vi "WriteToMeasArray.vi"(8 "error in (no error)":errorcluster, 10 "RoomAlert Device Reference":refnum<vi>, 11 "RoomAlert in":refnum<class "RoomAlert.lvclass">) -> (0 "error out":errorcluster, 3 "RoomAlert out":refnum<class "RoomAlert.lvclass">)   [LabVIEW 2018, in "SensorPlugins.lvlib" / "RoomAlert.lvclass"]
doc: "Updates to the measurement array all the values a user may measure from the RoomAlert."
uses:
  RoomAlert.lvclass
  TypeDefinitions/RoomAlertControls.ctl
panel:
  in  "Text Ring":u16(ring)
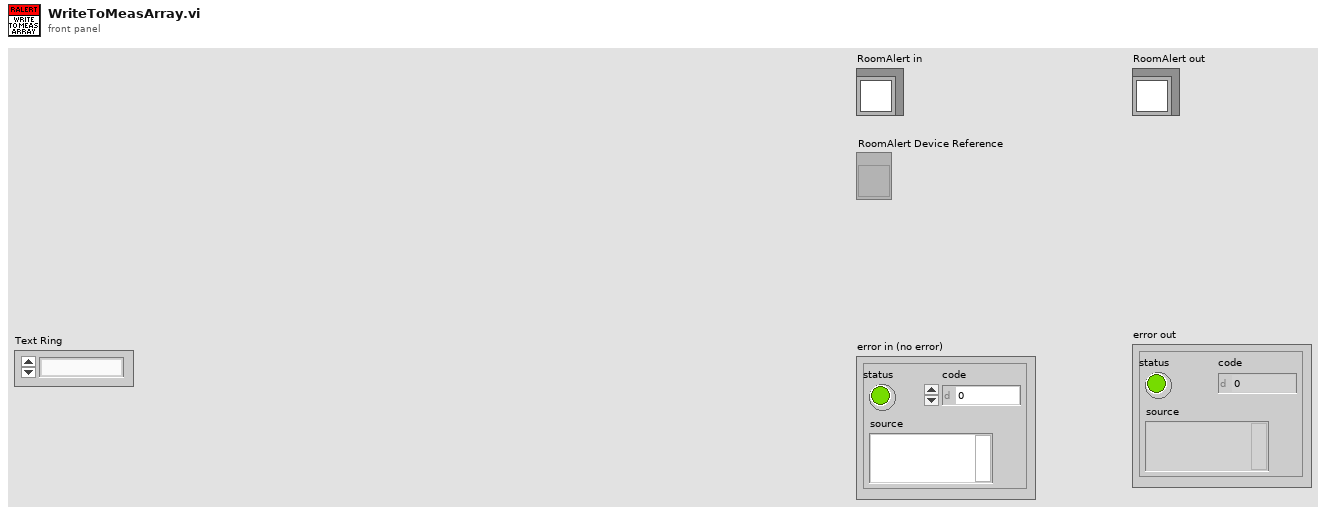
[diagram p1: front panel]
types:
  T1 = typedef "SensorPlugins.lvlib/RoomAlert.lvclass/MeasurementToRead.ctl" = cluster{"Type":string, "OID":string}[]
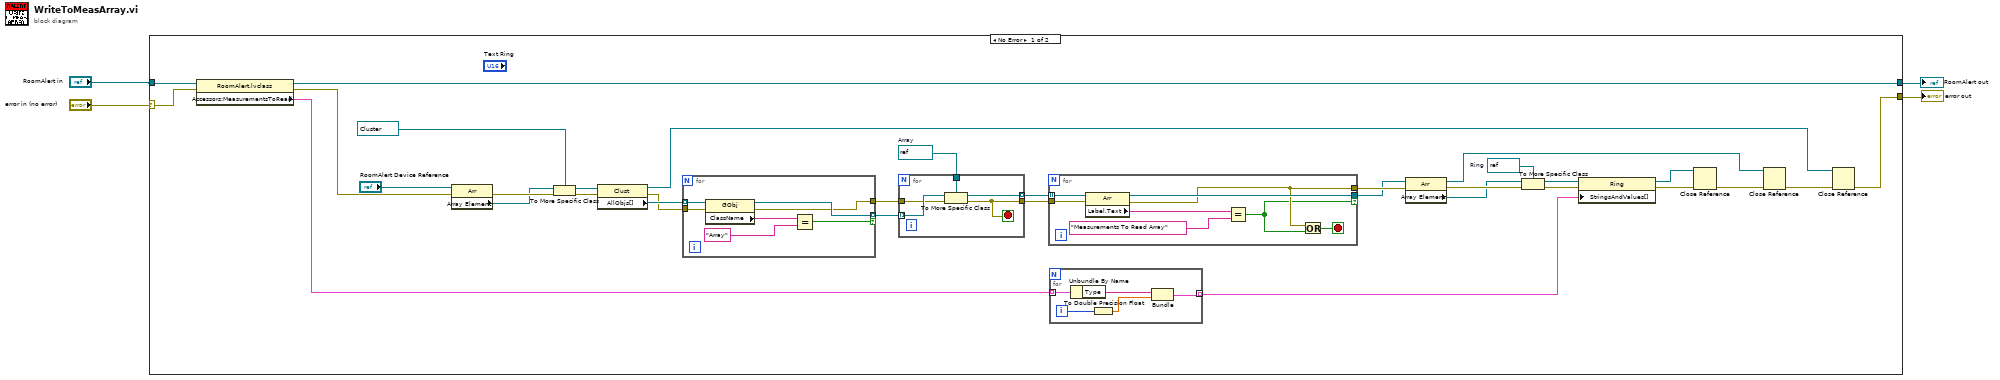
[diagram p0: block diagram]
diagram:
  n1 = case shown="No Error" "error in (no error)" {
    selector: "error in (no error)" -> [w36 w64]
    tunnel: [w19 w64] -> w1
    tunnel: [w35 w63] -> w2
    tunnel: "RoomAlert in" -> [w37 w63]
    frame No Error {
      w28 = refnum<vi> refnum  # Ring
      w8 = refnum<vi> refnum  # Array
      n2 = property class="RoomAlert.lvclass"(reference=w37, error in=w36) -> (reference out=w35:refnum<class "RoomAlert.lvclass">, error out=w34:errorcluster, "Accessors:MeasurementsToRead"=w14:T1)
      n3 = property class="Arr"(reference="RoomAlert Device Reference", error in=w34) -> (error out=w33:errorcluster, "Array Element"=w32:refnum<vi>)  [unwired: 1 out]
      n4 = To More Specific Class(target class=refnum<vi> refnum ("Text Ring"), reference=w32, error in=w33) -> (specific class reference=w29:refnum<vi>, error out=w30:errorcluster)
      n5 = property class="Clust"(reference=w29, error in=w30) -> (reference out=w16:refnum<vi>, error out=w11:errorcluster, "AllObjs[]"=w12:refnum<vi>[])
      n6 = for {
        tunnel: w12 -> [w44] mode=indexing
        tunnel: [w43] -> w9 mode=indexing if=w40
        tunnel: w11 -> [w41]
        tunnel: [w39] -> w10
        n7 = property class="GObj"(reference=w44, error in=w41) -> (reference out=w43:refnum<vi>, error out=w39:errorcluster, "ClassName"=w38:string)
        n8 = Equal?(x=w38, y="Array" ("ClassName")) -> (x = y?=w40:bool)
      }
      n9 = for {
        tunnel: w10 -> [w52]
        tunnel: w9 -> [w53] mode=indexing
        tunnel: w8 -> [w54]
        tunnel: [w51] -> w7 mode=indexing
        tunnel: [w50] -> w6
        stop <- w50 stop-if-true
        n10 = To More Specific Class(target class=w54, reference=w53, error in=w52) -> (specific class reference=w51:refnum<vi>, error out=w50:errorcluster)
      }
      n11 = for {
        tunnel: w7 -> [w62] mode=indexing
        tunnel: [w61] -> w15 if=w55
        tunnel: w6 -> [w59]
        tunnel: [w57] -> w17
        stop <- w58 stop-if-true
        n12 = property class="Arr"(reference=w62, error in=w59) -> (reference out=w61:refnum<vi>, error out=w57:errorcluster, "Label.Text"=w56:string)
        n13 = Equal?(x=w56, y="Measurements To Read Array" ("ClassName")) -> (x = y?=w55:bool)
        n14 = Or(x=w57, y=w55) -> (x .or. y?=w58:bool)
      }
      n15 = for {
        tunnel: w14 -> [w49] mode=indexing
        tunnel: [w45] -> w13 mode=indexing
        i -> [w48]
        n16 = Unbundle By Name(w49) -> ("Type"=w47:string)
        n17 = To Double Precision Float(number=w48) -> (double precision float=w46:dbl)
        n18 = Bundle("Type"=w47, w46) -> (w45:cluster{"Type":string, dbl})  [unwired: 1 in]
      }
      n19 = property class="Arr"(reference=w15, error in=w17) -> (reference out=w18:refnum<vi>, error out=w27:errorcluster, "Array Element"=w26:refnum<vi>)
      n20 = To More Specific Class(target class=w28, reference=w26, error in=w27) -> (specific class reference=w24:refnum<vi>, error out=w25:errorcluster)
      n21 = property class="Ring"(reference=w24, error in=w25, "StringsAndValues[]"=w13) -> (reference out=w22:refnum<vi>, error out=w23:errorcluster)
      n22 = Close Reference(reference=w22, error in (no error)=w23) -> (error out=w21:errorcluster)
      n23 = Close Reference(reference=w18, error in (no error)=w21) -> (error out=w20:errorcluster)
      n24 = Close Reference(reference=w16, error in (no error)=w20) -> (error out=w19:errorcluster)
    }
    frame Error {
    }
  }
  "error out" <- w1
  "RoomAlert out" <- w2
